vi "Write DQMH Modules.vi"(8 "error in (no error)":errorcluster, 10 "DQMH Modules":refnum<class "Dqmh Module.lvclass">[](array[class]), 11 "Dqmh Modules Overview in":refnum<class "Dqmh Modules Overview.lvclass">) -> (0 "error out":errorcluster, 3 "Dqmh Modules Overview out":refnum<class "Dqmh Modules Overview.lvclass">)   [LabVIEW 2021, in "TAF Proj Document Type.lvlib" / "Dqmh Modules Overview.lvclass"]
uses:
  <vilib>/Wovalab/AntiDoc/Document Type/Add-ons/LabVIEW TAF Project/Dqmh Modules Overview/Dqmh Modules Overview.lvclass
  <vilib>/Wovalab/AntiDoc/Document Type/Add-ons/LabVIEW TAF Project/Dqmh Module/Dqmh Module.lvclass
  <vilib>/Wovalab/AntiDoc/Document Type/Add-ons/LabVIEW TAF Project/Dqmh Modules Overview/Dqmh Modules Overview.lvclass/Dqmh Modules Overview.ctl
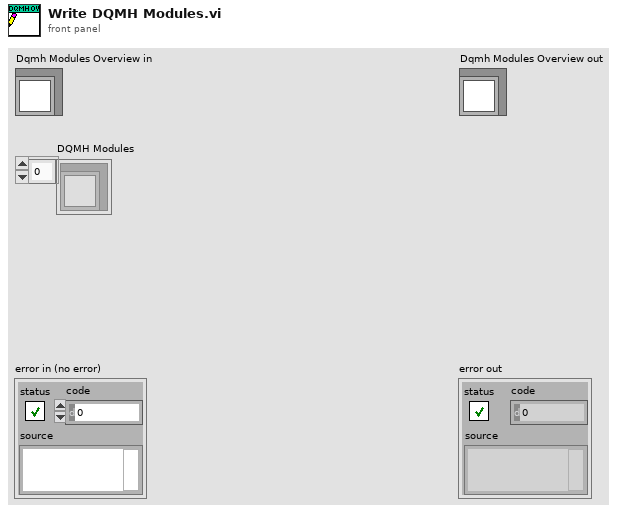
[diagram p1: front panel]
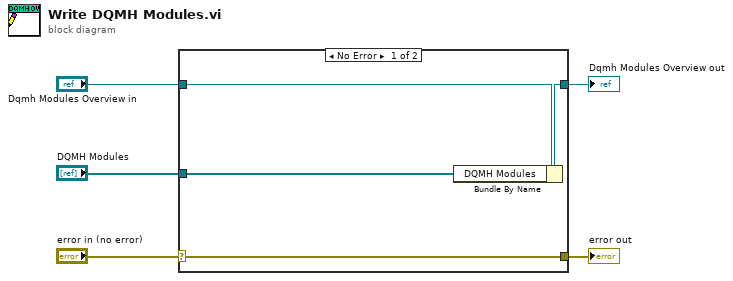
[diagram p0: block diagram]
diagram:
  n1 = case shown="No Error" "error in (no error)" {
    selector: "error in (no error)" -> [w9 w10]
    tunnel: [w9 w10] -> w4
    tunnel: [w7 w11] -> w2
    tunnel: "Dqmh Modules Overview in" -> [w8 w11]
    tunnel: "DQMH Modules" -> [w6 _]
    frame No Error {
      n2 = Bundle By Name(cluster=w8, "DQMH Modules"=w6) -> (w7:refnum<class "Dqmh Modules Overview.lvclass">)
    }
    frame Error {
    }
  }
  "error out" <- w4
  "Dqmh Modules Overview out" <- w2
